vi "GetAllDepsUsingLVProj.vi"(8 "error in (no error)":errorcluster, 11 "Project Path":path=path "E:/sw-deps-monitor/Source/BuildSpecs/Modules/ModuleA.lvproj") -> (0 "error out":errorcluster, 3 "Actual Dependencies":string[](array[string]))   [LabVIEW 2019, in "Hawkeye.lvlib"]
uses:
  Hawkeye.lvlib
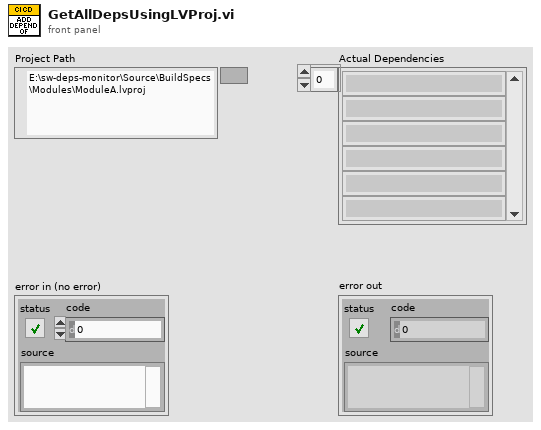
[diagram p1: front panel]
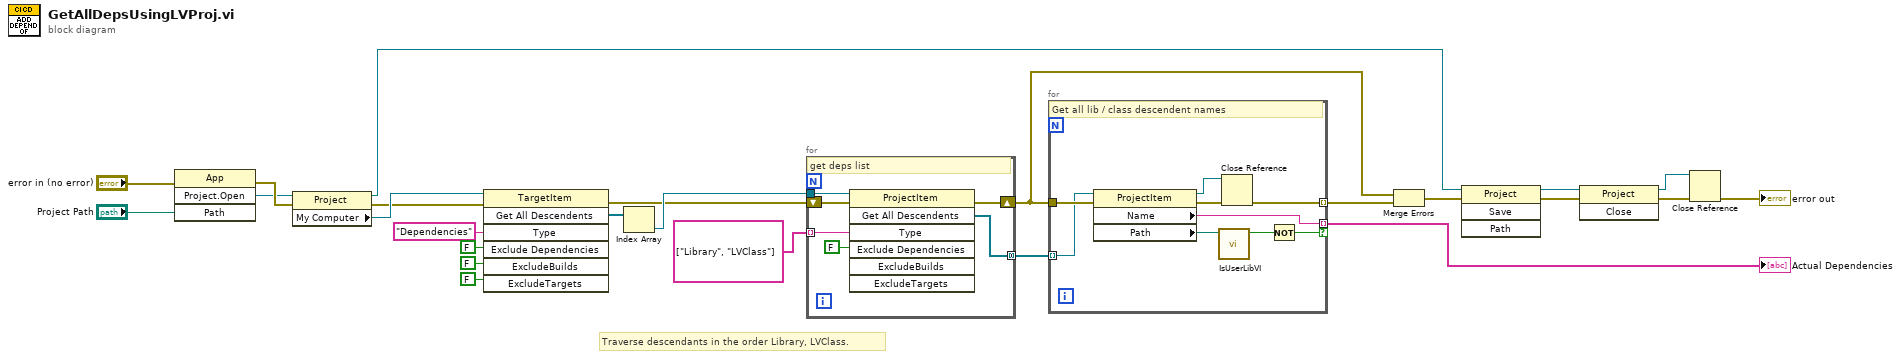
[diagram p0: block diagram]
diagram:
  # "Traverse descendants in the order Library, LVClass."
  n1 = invoke class="App" method="Project.Open"(error in="error in (no error)", "Path"="Project Path") -> (error out=w21:errorcluster, "Project:Open"=w20:refnum<vi>)  [unwired: 2 in, 2 out]
  n2 = property class="Project"(reference=w20, error in=w21) -> (reference out=w8:refnum<vi>, error out=w11:errorcluster, "My Computer"=w15:refnum<vi>)
  n3 = invoke class="TargetItem" method="Get All Descendents"(reference=w15, error in=w11, "Type"="Dependencies", "Exclude Dependencies"=FALSE ("ExcludeDependencies"), "ExcludeBuilds"=FALSE, "ExcludeTargets"=FALSE) -> (error out=w10:errorcluster, "All Descendents"=w13:refnum<vi>[])  [unwired: 1 in, 5 out]
  n4 = Index Array(array=w13) -> (element=w12:refnum<vi>)  [unwired: 1 in]
  n5 = for {
    tunnel: w12 -> [w30]
    tunnel: [w27] -> w7 mode=concatenating
    shift-right: [w28] -> w1
    shift-left: w10 -> [w29]
    tunnel: string[] ["Library", "LVClass"] ("Type") -> [w26] mode=indexing
    # "get deps list"
    n6 = invoke class="ProjectItem" method="Get All Descendents"(reference=w30, error in=w29, "Type"=w26, "Exclude Dependencies"=FALSE ("ExcludeDependencies")) -> (error out=w28:errorcluster, "All Descendents"=w27:refnum<vi>[])  [unwired: 3 in, 5 out]
  }
  n7 = for {
    tunnel: w1 -> [w40]
    tunnel: w7 -> [w39] mode=indexing
    tunnel: [w36] -> w19 mode=indexing
    tunnel: [w34] -> w23 mode=indexing if=w32
    # "Get all lib / class descendent names"
    n8 = property class="ProjectItem"(reference=w39, error in=w40) -> (reference out=w35:refnum<vi>, error out=w38:errorcluster, "Name"=w34:string, "Path"=w37:path)
    n9 = call "IsUserLibVI.vi"("ItemPath"=w37) -> ("IsUserLibVI?"=w33:bool)  [unwired: 10 in]
    n10 = Close Reference(reference=w35, error in (no error)=w38) -> (error out=w36:errorcluster)
    n11 = Not(x=w33) -> (.not. x?=w32:bool)
  }
  "Actual Dependencies" <- w23
  n12 = Merge Errors(w1, w19) -> (w9:errorcluster)
  n13 = invoke class="Project" method="Save"(reference=w8, error in=w9) -> (reference out=w5:refnum<vi>, error out=w3:errorcluster)  [unwired: 2 in, 2 out]
  n14 = invoke class="Project" method="Close"(reference=w5, error in=w3) -> (reference out=w4:refnum<vi>, error out=w2:errorcluster)  [unwired: 1 in, 1 out]
  n15 = Close Reference(reference=w4, error in (no error)=w2) -> (error out=→"error out":errorcluster)
